vi "Probe Test.vi"   [LabVIEW 2015, in "ByRef Variant Repository.lvlib"]
uses:
  ByRef Variant Repository.lvlib
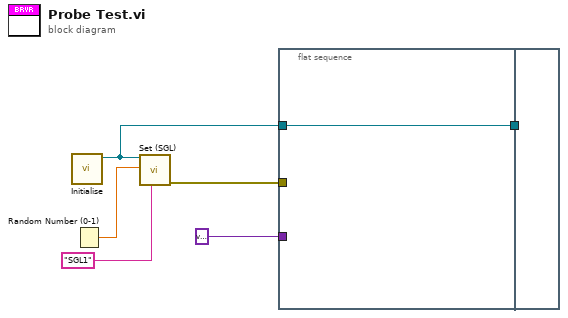
[diagram p0: block diagram]
diagram:
  n1 = call "Initialise.vi"() -> ("ByRef Variant Repsitory out"=w5:refnum<data-value>)  [unwired: 9 in, 1 out]
  n2 = Random Number (0-1)() -> (number: 0 to 1=w1:dbl)
  n3 = call "Set (SGL).vi"("Tag"="SGL1", "Value"=w1, "ByRef Variant Repsitory in"=w5) -> ("error out"=w6:errorcluster)  [unwired: 7 in]
  n4 = flat-sequence {
    tunnel: w6 -> [_]
    tunnel: w5 -> [w7]
    tunnel: [w7] -> w4
    tunnel: variant -> [_]
    tunnel: w4 -> [_]
    frame #0 {
    }
    frame #1 {
    }
  }
